vi "Adv_SetROI.vi"(8 "error in (no error)":errorcluster, 10 "ROI":T1(ring), 11 "LightField Automation in":refnum<class "LightField Automation.lvclass">) -> (0 "error out":errorcluster, 3 "LightField Automation out":refnum<class "LightField Automation.lvclass">)   [LabVIEW 2019, in "LightField Automation.lvclass"]
uses:
  LightField Automation.lvclass
  LightField Automation.lvclass/LightField Automation.ctl
  C:/Program Files/Princeton Instruments/LightField/AddInViews/PrincetonInstruments.LightFieldViewV3.dll
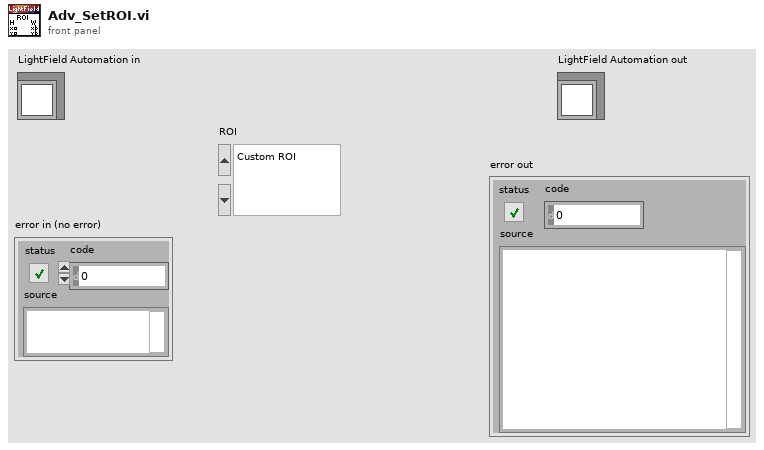
[diagram p1: front panel]
types:
  T1 = enum16{"Custom ROI", "Full sensor", "Binned full sensor"}
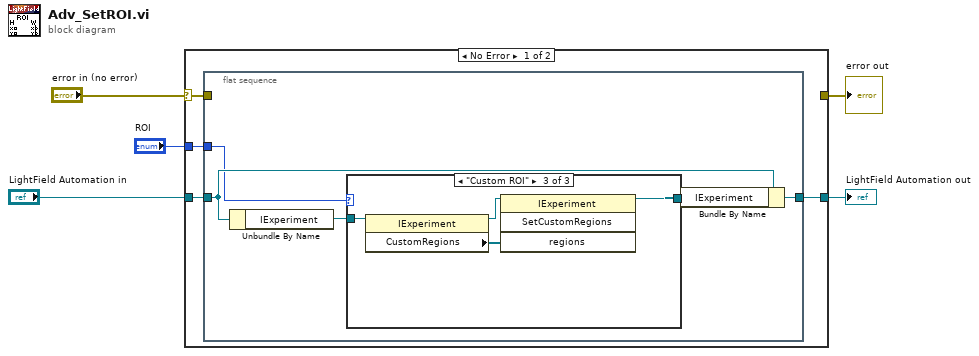
[diagram p0: block diagram]
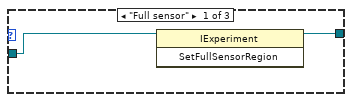
[diagram p2: hidden frame]
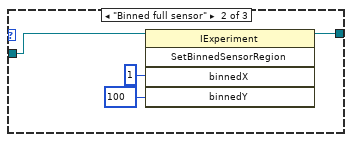
[diagram p3: hidden frame]
diagram:
  n1 = case shown="No Error" "error in (no error)" {
    selector: "error in (no error)" -> [w9 w26]
    tunnel: [_ w26] -> w4
    tunnel: "LightField Automation in" -> [w8 w25]
    tunnel: [w7 w25] -> w2
    tunnel: "ROI" -> [w6 _]
    frame No Error {
      n2 = flat-sequence {
        tunnel: w9 -> [_]
        tunnel: w8 -> [w13]
        tunnel: [w12] -> w7
        tunnel: w6 -> [w10]
        frame #0 {
          n3 = Unbundle By Name(w13) -> ("IExperiment"=w11:refnum<k24>)
          n4 = case shown="\"Custom ROI\"" w10 {
            tunnel: [w16 w20 w24] -> w14
            tunnel: w11 -> [w15 w19 w22]
            frame "Full sensor" {
              n5 = invoke class="IExperiment" method="SetFullSensorRegion"(reference=w15) -> (reference out=w16:refnum<k24>)  [unwired: 2 in, 2 out]
            }
            frame "Binned full sensor" {
              n6 = invoke class="IExperiment" method="SetBinnedSensorRegion"(reference=w19, "binnedX"=1, "binnedY"=100) -> (reference out=w20:refnum<k24>)  [unwired: 2 in, 4 out]
            }
            frame "Custom ROI" {
              n7 = property class="IExperiment"(reference=w22) -> (reference out=w21:refnum<k24>, "CustomRegions"=w23:refnum<k24>[])  [unwired: 1 in, 1 out]
              n8 = invoke class="IExperiment" method="SetCustomRegions"(reference=w21, "regions"=w23) -> (reference out=w24:refnum<k24>)  [unwired: 2 in, 3 out]
            }
          }
          n9 = Bundle By Name(cluster=w13, "IExperiment"=w14) -> (w12:refnum<class "LightField Automation.lvclass">)
        }
      }
    }
    frame Error {
    }
  }
  "LightField Automation out" <- w2
  "error out" <- w4
